vi "AP_project_calibration_step_by_step.vi"() -> ()   [LabVIEW 2019]
uses:
  <vilib>/userDefined/High Color/IMAQdx.ctl
  <vilib>/vision/driver/IMAQdx.llb/IMAQdx Acquisition Mode.ctl
  <vilib>/vision/Calibration.llb/Distortion Model.ctl
  <vilib>/vision/Calibration.llb/Distortion Model Types.ctl
  <vilib>/vision/driver/NI_Vision_Acquisition_Software.lvlib
  <vilib>/vision/NI_Vision_Development_Module.lvlib
panel:
  in  "Range":cluster{"Lower value":sgl, "Upper value":sgl}={"Lower value"=128.0, "Upper value"=255.0} {"Upper value" format="%.2f"; "Lower value" format="%.2f"}
  out "Calibration Image Path":string
  in  "Recalibrate Camera":bool
  out "Calibration Error Statistics":T1
  out "Processed Image":T2(plugin-control)
  in  "Number of Frames to Get":u32
  in  "IMAQdx Session":T3="cam0"
  out "Acquired Image":T2(plugin-control)
  out "height":dbl
  out "width":dbl
  in  "Display Index":i32
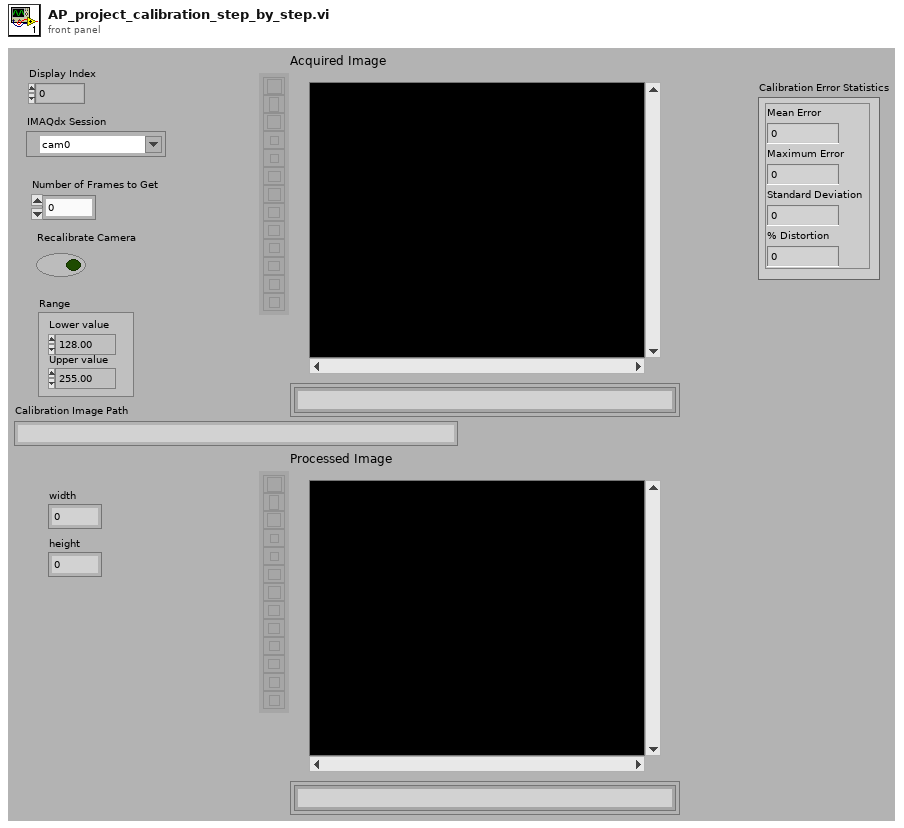
[diagram p1: front panel]
types:
  T1 = cluster{"Mean Error":dbl, "Maximum Error":dbl, "Standard Deviation":dbl, "% Distortion":dbl}
  T2 = typedef "IMAQ Image.ctl" = refnum<image>
  T3 = typedef "IMAQdx.ctl" = refnum<k21>
  T4 = typedef "Image Unit" = enum32{"Undefined", "Angström", "Micrometer", "Millimeter", "Centimeter", "Meter", "Kilometer", "Microinch", "Inch", "Feet", "Nautical miles", "Standard miles", "Steps"}
  T5 = typedef "LVAllMonitorsDisplayTypeDef.ctl" = cluster{"Bounds":cluster{"Left":i16, "Top":i16, "Right":i16, "Bottom":i16}, "Depth":i16}[]
  T6 = cluster{"Bounds":cluster{"Left":i16, "Top":i16, "Right":i16, "Bottom":i16}, "Depth":i16}
  T7 = typedef "Image Type" = u32
  T8 = typedef "NI_Vision_Acquisition_Software.lvlib/IMAQdx Acquisition Mode.ctl" = enum32{"One Shot", "Continuous"}
  T9 = typedef "Distortion Model.ctl" = cluster{"Distortion Model":T10, "Polynomial Model Setup":cluster{"Radial Coefficient":u32, "Tangential Coefficients ":bool}}
  T10 = typedef "Distortion Model Types.ctl" = i32
  T11 = typedef "Particle Parameters" = i32
  T12 = cluster{"Measurement Parameter":T11, "Range Lower Value":dbl, "Range Upper Value":dbl, "Range":bool, "Measurement Type":bool}[]
  T13 = typedef "Calibration Reference Points.ctl" = cluster{"Pixel Coordinates":cluster{"X":dbl, "Y":dbl}[], "Real World Coordinates":cluster{"X":dbl, "Y":dbl}[], "Unit":T4, "Image Size":cluster{"X":u32, "Y":u32}}
  T14 = typedef "Error Statistics.ctl" = cluster{"Mean Error":dbl, "Maximum Error":dbl, "Standard Deviation":dbl, "% Distortion":dbl}
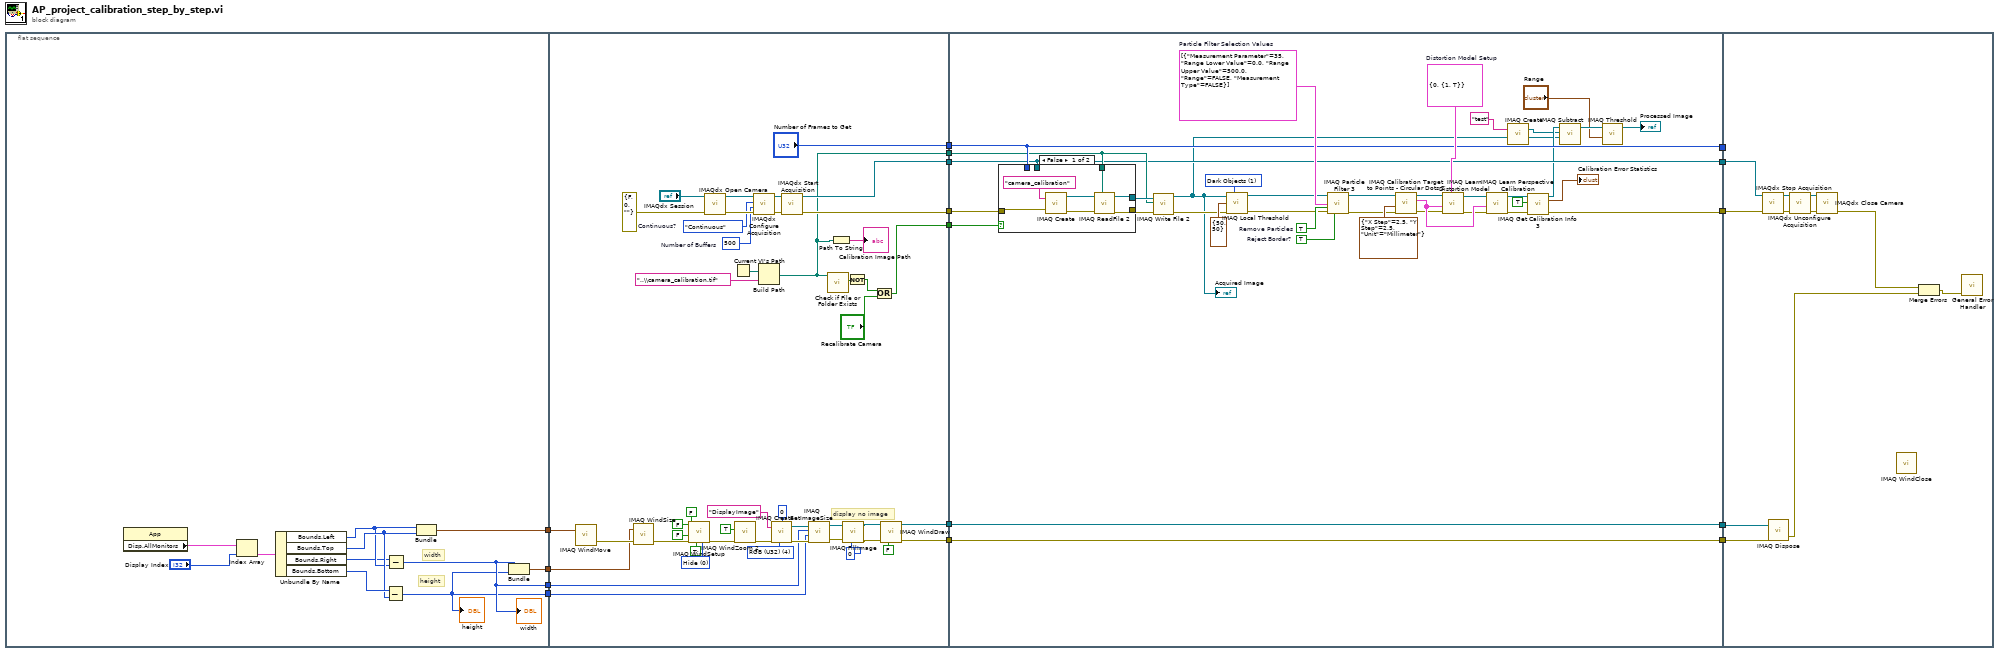
[diagram p0: block diagram]
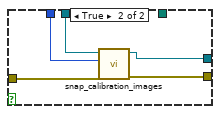
[diagram p2: hidden frame]
diagram:
  n1 = flat-sequence {
    tunnel: [w20] -> w16
    tunnel: [w19] -> w15
    tunnel: [w18] -> w12
    tunnel: [w17] -> w11
    tunnel: w16 -> [w70]
    tunnel: w15 -> [w68]
    tunnel: [w55] -> w14
    tunnel: w12 -> [w47]
    tunnel: w11 -> [w46]
    tunnel: [w39] -> w8
    tunnel: [w38] -> w7
    tunnel: ["Number of Frames to Get"] -> w5
    tunnel: [w36] -> w4
    tunnel: [w33] -> w3
    tunnel: [w29] -> w2
    tunnel: w14 -> [w88]
    tunnel: [w83] -> w13
    tunnel: [w111] -> w10
    tunnel: [w110] -> w9
    tunnel: w8 -> [w111]
    tunnel: w7 -> [w110]
    tunnel: [w87] -> w6
    tunnel: w5 -> [w87]
    tunnel: w4 -> [w83]
    tunnel: w3 -> [w89]
    tunnel: w2 -> [w85]
    tunnel: [w81] -> w1
    tunnel: w13 -> [w128]
    tunnel: w10 -> [w126]
    tunnel: w9 -> [w125]
    tunnel: w6 -> [_]
    tunnel: w1 -> [w129]
    frame #0 {
      # "height"
      # "width"
      n2 = property class="App"() -> ("Disp.AllMonitors"=w23:T5)  [unwired: 2 in, 2 out]
      n3 = Index Array(array=w23, index="Display Index") -> (element=w22:T6)
      n4 = Unbundle By Name(w22) -> ("Bounds.Left"=w25:i16, "Bounds.Top"=w26:i16, "Bounds.Right"=w24:i16, "Bounds.Bottom"=w27:i16)
      n5 = Subtract(x=w27, y=w26) -> (x-y=w17:i16)
      "height" <- w17
      n6 = Subtract(x=w24, y=w25) -> (x-y=w18:i16)
      "width" <- w18
      n7 = Bundle("Left"=w25, "Top"=w26) -> (w19:cluster{"Left":i16, "Top":i16})  [unwired: 1 in]
      n8 = Bundle(w18, w17) -> (w20:cluster{i16, i16})  [unwired: 1 in]
    }
    frame #1 {
      w48 = T7 4 items=["Grayscale (U8)", "Grayscale (I16)", "Grayscale (SGL)", "Complex (CSG)", "RGB (U32)", "HSL (U32)", "RGB (U64)"] ("Image Type")
      w57 = u32 500  # Number of Buffers
      w56 = IMAQdx_Acquisition_Mode."Continuous"  # Continuous?
      w67 = 0 items=["Hide", "Show", "No change"] ("Scrollbars (No change)")
      # "display no image"
      n9 = call "IMAQ WindMove"("Coordinates (screen)"=w68) -> ("error out"=w72:errorcluster)  [unwired: 4 in, 1 out]
      n10 = call "IMAQ WindSize"("error in (no error)"=w72, "Width & Height"=w70) -> ("error out"=w73:errorcluster)  [unwired: 4 in, 2 out]
      n11 = call "IMAQ WindSetup"("Scrollbars (No change)"=w67, "Window is floating? (No)"=TRUE, "error in (no error)"=w73, "Window has title bar? (Yes)"=FALSE, "Window can close? (Yes)"=FALSE, "Window can grow? (Yes)"=FALSE) -> ("error out"=w71:errorcluster)  [unwired: 5 in]
      n12 = call <vilib>:"IMAQdx Open Camera.vi"("error in"=errorcluster {"status"=FALSE, "code"=0, "source"=""}, "Session In"="IMAQdx Session") -> ("error out"=w61:errorcluster, "Session Out"=w62:T3)  [unwired: 8 in]
      n13 = Current VI's Path() -> (path=w35:path)
      n14 = call "IMAQ WindZoom 2"("error in (no error)"=w71, "Zoom to Fit? (False)"=TRUE ("Zoom to Fit? (T)")) -> ("error out"=w51:errorcluster)  [unwired: 6 in, 3 out]
      n15 = call <vilib>:"IMAQdx Configure Acquisition.vi"("error in"=w61, "Number of Buffers"=w57, "Continuous?"=w56, "Session In"=w62) -> ("error out"=w60:errorcluster, "Session Out"=w58:T3)  [unwired: 6 in]
      n16 = Build Path(base path=w35, name or relative path="..\\camera_calibration.tif") -> (appended path=w29:path)
      n17 = call "IMAQ Create"("Border Size"=0, "Image Name"="DisplayImage", "Image Type"=w48, "error in (no error)"=w51) -> ("New Image"=w52:T2, "error out"=w53:errorcluster)  [unwired: 1 in]
      n18 = call <vilib>:"IMAQdx Start Acquisition.vi"("error in"=w60, "Session In"=w58) -> ("error out"=w55:errorcluster, "Session Out"=w36:T3)  [unwired: 8 in]
      n19 = call "IMAQ SetImageSize"("error in (no error)"=w53, "Y Resolution"=w46, "X Resolution"=w47, "Image"=w52) -> ("error out"=w40:errorcluster, "Image Out"=w41:T2)  [unwired: 1 in]
      n20 = call <vilib>:"Check if File or Folder Exists.vi"("path"=w29) -> ("file or folder exists?"=w31:bool)  [unwired: 8 in, 2 out]
      n21 = Path To String(path=w29) -> (string=→"Calibration Image Path":string)
      n22 = call "IMAQ FillImage"("Color Pixel Value"=0, "error in (no error)"=w40, "Image"=w41) -> ("error out"=w45:errorcluster, "Image Out"=w44:T2)  [unwired: 7 in]
      n23 = Not(x=w31) -> (.not. x?=w30:bool)
      n24 = Or(x=w30, y="Recalibrate Camera") -> (x .or. y?=w33:bool)
      n25 = call "IMAQ WindDraw"("Resize to Image Size? (Y)"=FALSE, "error in (no error)"=w45, "Image"=w44) -> ("error out"=w38:errorcluster, "Image Out (duplicate)"=w39:T2)  [unwired: 7 in]
    }
    frame #2 {
      w100 = T9 {"Distortion Model"=0, "Polynomial Model Setup"={"Radial Coefficient"=1, "Tangential Coefficients "=TRUE}}  # Distortion Model Setup
      w101 = T12 [{"Measurement Parameter"=35, "Range Lower Value"=0.0, "Range Upper Value"=500.0, "Range"=FALSE, "Measurement Type"=FALSE}]  # Particle Filter Selection Values
      w103 = TRUE  # Remove Particles
      w102 = TRUE  # Reject Border?
      w108 = u32 1 items=["Bright Objects", "Dark Objects"] ("Look For (Bright Objects)")
      n26 = case shown="False" w89 {
        tunnel: w88 -> [w117 w123]
        tunnel: [w114 w122] -> w86
        tunnel: w87 -> [_ w121]
        tunnel: [w115 w120] -> w84
        tunnel: w85 -> [w112 _]
        tunnel: w83 -> [_ w119]
        frame False {
          n27 = call "IMAQ Create"("Image Name"="camera_calibration", "error in (no error)"=w117) -> ("New Image"=w113:T2, "error out"=w116:errorcluster)  [unwired: 2 in, 1 out]
          n28 = call "IMAQ ReadFile 2"("File Path"=w112, "error in (no error)"=w116, "Image"=w113) -> ("error out"=w115:errorcluster, "Image Out"=w114:T2)  [unwired: 4 in, 3 out]
        }
        frame True {
          n29 = call "snap_calibration_images.vi"("error in (no error)"=w123, "Number of Frames to Get"=w121, "Session In"=w119) -> ("error out"=w120:errorcluster, "Image Out"=w122:T2)  [unwired: 7 in]
        }
      }
      n30 = call-poly "IMAQ Write File 2"("error in (no error)"=w84, "File Path"=w85, "Image"=w86) -> ("error out"=w82:errorcluster, "Image Out (duplicate)"=w76:T2)  [unwired: 7 in]
      "Acquired Image" <- w76
      n31 = call "IMAQ Local Threshold"("Image Src"=w76, "Look For (Bright Objects)"=w108, "Window Size (32x32)"=cluster{"SizeX":i32, "SizeY":i32} {"SizeX"=50, "SizeY"=50}, "error in (no error)"=w82) -> ("Image Dst Out"=w90:T2, "error out"=w99:errorcluster)  [unwired: 5 in, 5 out]
      n32 = call "IMAQ Particle Filter 3"("Image Src"=w90, "Selection Values"=w101, "Keep/Remove Particles (F)"=w103, "error in (no error)"=w99, "Reject Border? (F)"=w102) -> ("Image Dst Out"=w91:T2, "error out"=w98:errorcluster)  [unwired: 4 in, 5 out]
      n33 = call "IMAQ Calibration Target to Points - Circular Dots 2"("error in (no error)"=w98, "Grid Descriptor"=cluster{"X Step":sgl, "Y Step":sgl, "Unit":T4} {"X Step"=2.5, "Y Step"=2.5, "Unit"=enum."Millimeter"}, "Target Image"=w91) -> ("error out"=w97:errorcluster, "Reference Points"=w105:T13, "Target Image (dup)"=w107:T2)  [unwired: 6 in]
      n34 = call "IMAQ Learn Distortion Model"("Distortion Model Setup"=w100, "error in (no error)"=w97, "Reference Points"=w105, "Calibration Template Image"=w107) -> ("error out"=w96:errorcluster, "Calibration Template Image Out"=w106:T2)  [unwired: 2 in, 4 out]
      n35 = call "IMAQ Learn Perspective Calibration"("error in (no error)"=w96, "Reference Points"=w105, "Calibration Template Image"=w106) -> ("error out"=w92:errorcluster, "Calibration Template Image Out"=w95:T2)  [unwired: 1 in, 6 out]
      n36 = call "IMAQ Create"("Image Name"="test") -> ("New Image"=w74:T2)  [unwired: 3 in, 2 out]
      n37 = call "IMAQ Get Calibration Info 3"("Calibration Template Image"=w95, "Return Error Information (False)"=TRUE, "error in (no error)"=w92) -> ("Calibration Template Image (duplicate)"=w77:T2, "Error Statistics"=→"Calibration Error Statistics":T14, "error out"=w81:errorcluster)  [unwired: 4 in, 6 out]
      n38 = call "IMAQ Subtract"("Image Src A"=w77, "Image Dst"=w74, "Image Src B"=w76) -> ("Image Dst Out"=w80:T2)  [unwired: 4 in, 1 out]
      n39 = call "IMAQ Threshold"("Range"="Range", "Image Src"=w80) -> ("Image Dst Out"=→"Processed Image":T2)  [unwired: 8 in, 1 out]
    }
    frame #3 {
      n40 = call <vilib>:"IMAQdx Stop Acquisition.vi"("error in"=w129, "Session In"=w128) -> ("error out"=w130:errorcluster, "Session Out"=w131:T3)  [unwired: 8 in]
      n41 = call "IMAQ Dispose"("Image"=w126, "error in (no error)"=w125) -> ("error out"=w124:errorcluster)  [unwired: 4 in]
      n42 = call <vilib>:"IMAQdx Unconfigure Acquisition.vi"("error in"=w130, "Session In"=w131) -> ("error out"=w133:errorcluster, "Session Out"=w132:T3)  [unwired: 8 in]
      n43 = call <vilib>:"IMAQdx Close Camera.vi"("error in"=w133, "Session In"=w132) -> ("error out"=w127:errorcluster)  [unwired: 9 in]
      n44 = call "IMAQ WindClose"() -> ()  [unwired: 6 in, 1 out]
      n45 = Merge Errors(w127, w124) -> (w134:errorcluster)
      n46 = call <vilib>:"General Error Handler.vi"("error in (no error)"=w134) -> ()  [unwired: 10 in, 5 out]
    }
  }
